vi "Generate JKISM Message Event.vi"(8 "error in (no error)":errorcluster, 10 "JKISM Message":string, 11 "Module":string) -> (0 "error out":errorcluster)   [LabVIEW 2017, in "JKISM Message Event.lvlib"]
uses:
  JKISM Message Event.lvlib
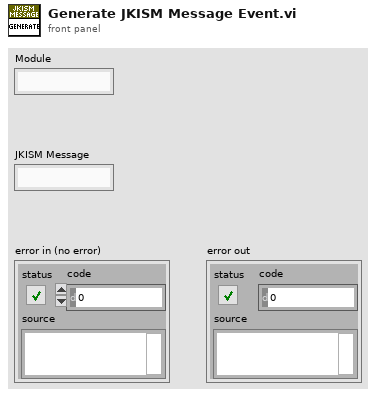
[diagram p1: front panel]
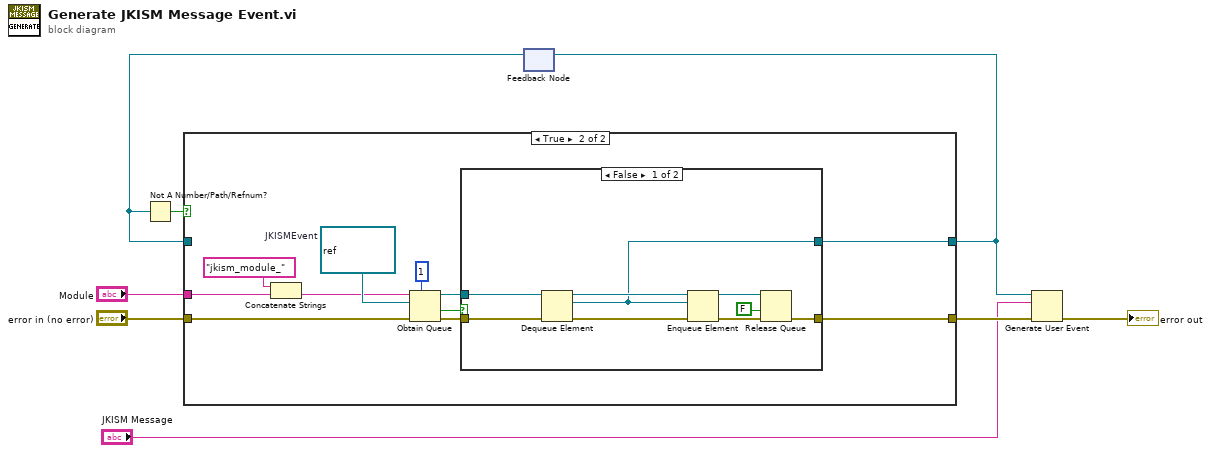
[diagram p0: block diagram]
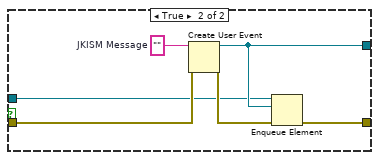
[diagram p3: hidden frame]
diagram:
  n1 = feedback #1() -> (w4:refnum<user-event>)  [unwired: 1 in]
  n2 = Not A Number/Path/Refnum?(number/path/refnum=w4) -> (NaN/Path/Refnum?=w5:bool)
  n3 = case shown="True" w5 {
    tunnel: "Module" -> [_ w21]
    tunnel: "error in (no error)" -> [w9 w20]
    tunnel: [w9 w11] -> w6
    tunnel: [w10 w12] -> w2
    tunnel: w4 -> [w10 _]
    frame False {
    }
    frame True {
      w16 = refnum<user-event> refnum  # JKISMEvent
      n4 = Concatenate Strings("jkism_module_" ("string"), w21) -> (w14:string)
      n5 = Obtain Queue(max queue size (-1, unlimited)=1, name (unnamed)=w14, element data type=w16, error in (no error)=w20) -> (queue out=w18:refnum<queue>, created new?=w15:bool, error out=w19:errorcluster)  [unwired: 1 in]
      n6 = case shown="False" w15 {
        tunnel: [w22 w36] -> w11
        tunnel: w19 -> [w30 w34]
        tunnel: [w26 w33] -> w12
        tunnel: w18 -> [w28 w32]
        frame False {
          n7 = Dequeue Element(queue=w28, error in (no error)=w30) -> (queue out=w27:refnum<queue>, element=w26:refnum<user-event>, error out=w29:errorcluster)  [unwired: 1 in, 1 out]
          n8 = Enqueue Element(queue=w27, element=w26, error in (no error)=w29) -> (queue out=w23:refnum<queue>, error out=w24:errorcluster)  [unwired: 1 in, 1 out]
          n9 = Release Queue(queue=w23, force destroy? (F)=FALSE, error in (no error)=w24) -> (error out=w22:errorcluster)  [unwired: 2 out]
        }
        frame True {
          w31 = ""  # JKISM Message
          n10 = Create User Event(user event datatype=w31, error in=w34) -> (user event=w33:refnum<user-event>, error out=w35:errorcluster)
          n11 = Enqueue Element(queue=w32, element=w33, error in (no error)=w35) -> (error out=w36:errorcluster)  [unwired: 1 in, 2 out]
        }
      }
    }
  }
  n12 = feedback-in #1(w2) -> ()
  n13 = Generate User Event(user event=w2, event data cluster="JKISM Message", error in=w6) -> (error out=→"error out":errorcluster)  [unwired: 1 in, 1 out]
